vi "Choose Elevator Load Position.vi"(9 "Have Trashcan?":bool, 10 "Presets":T1, 11 "Command":T2) -> (3 "Elevator Position":dbl)   [LabVIEW 2014]
uses:
  Elevator Command.ctl
  Common Code/Elevator Presets.ctl
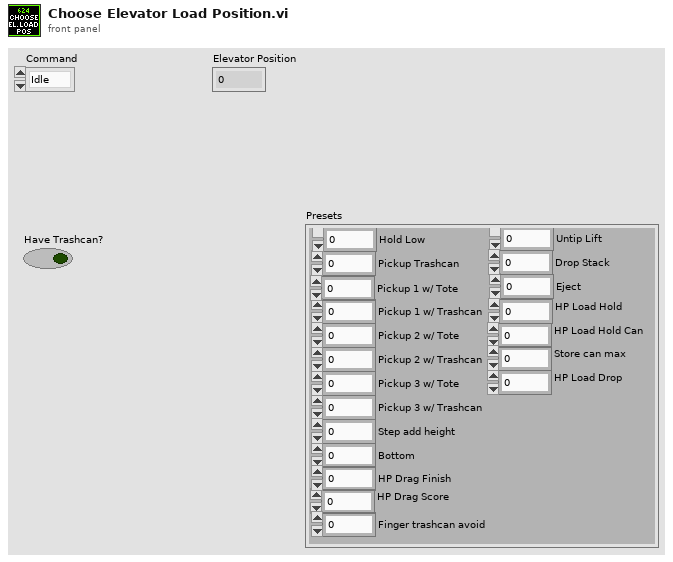
[diagram p1: front panel]
types:
  T1 = typedef "Elevator Presets.ctl" = cluster{"Pickup 2 w/ Tote":sgl, "Pickup 2 w/ Trashcan":sgl, "Pickup 3 w/ Tote":sgl, "Pickup 3 w/ Trashcan":sgl, "Bottom":sgl, "Pickup 1 w/ Tote":sgl, "Pickup Trashcan":sgl, "Pickup 1 w/ Trashcan":sgl, "Eject":sgl, "Hold Low":sgl, "Step add height":sgl, "Untip Lift":dbl, "Drop Stack":dbl, "HP Load Hold":dbl, "HP Load Drop":dbl, "HP Load Hold Can":dbl, "Store can max":dbl, "HP Drag Score":dbl, "HP Drag Finish":dbl, "Finger trashcan avoid":dbl}
  T2 = typedef "Elevator Command.ctl" = enum16{"Idle", "Load 1", "Load 2", "Load 3", "Drop Stack", "Eject Stack", "Untip Trashcan", "Load Trashcan", "HP Load", "HP Score"}
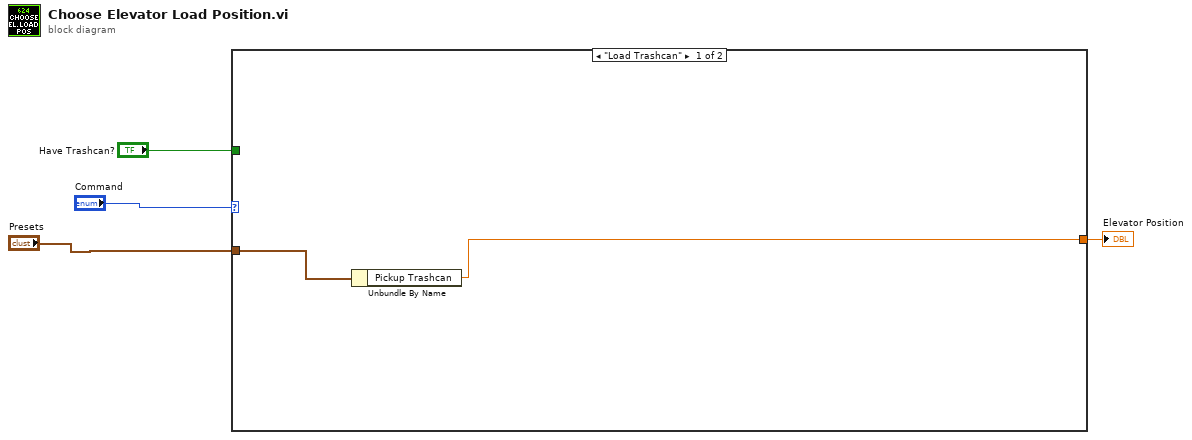
[diagram p0: block diagram]
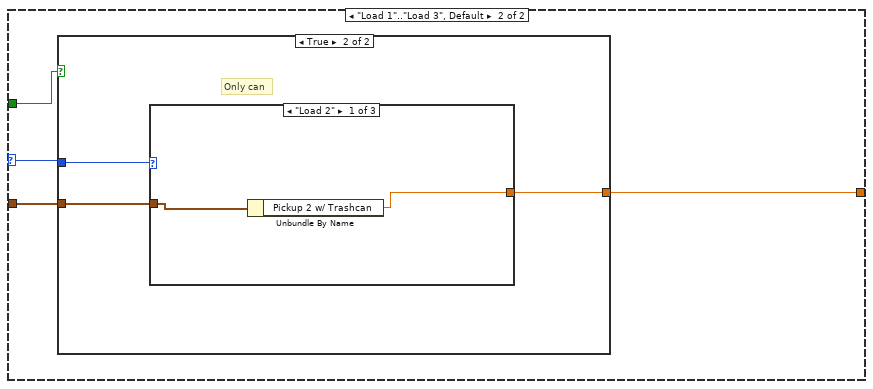
[diagram p2: hidden frame]
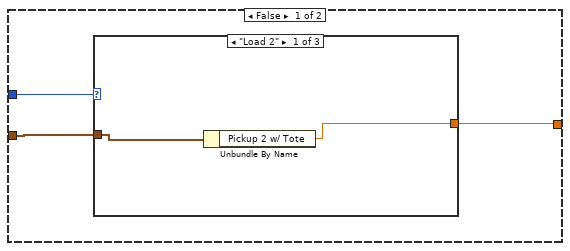
[diagram p3: hidden frame]
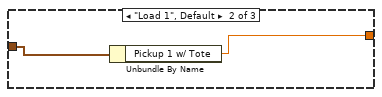
[diagram p4: hidden frame]
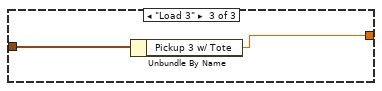
[diagram p5: hidden frame]
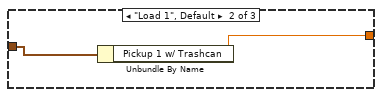
[diagram p6: hidden frame]
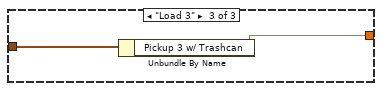
[diagram p7: hidden frame]
diagram:
  n1 = case shown="\"Load Trashcan\"" "Command" {
    selector: "Command" -> [_ w9]
    tunnel: "Presets" -> [w6 w10]
    tunnel: [w5 w8] -> w3
    tunnel: "Have Trashcan?" -> [_ w7]
    frame "Load Trashcan" {
      n2 = Unbundle By Name(w6) -> ("Pickup Trashcan"=w5:sgl)
    }
    frame "Load 1".."Load 3", Default {
      n3 = case shown="True" w7 {
        tunnel: w10 -> [w13 w22]
        tunnel: w9 -> [w12 w21]
        tunnel: [w11 w20] -> w8
        frame False {
          n4 = case shown="\"Load 2\"" w12 {
            tunnel: w13 -> [w15 w17 w19]
            tunnel: [w14 w16 w18] -> w11
            frame "Load 2" {
              n5 = Unbundle By Name(w15) -> ("Pickup 2 w/ Tote"=w14:sgl)
            }
            frame "Load 1", Default {
              n6 = Unbundle By Name(w17) -> ("Pickup 1 w/ Tote"=w16:sgl)
            }
            frame "Load 3" {
              n7 = Unbundle By Name(w19) -> ("Pickup 3 w/ Tote"=w18:sgl)
            }
          }
        }
        frame True {
          # "Only can"
          n8 = case shown="\"Load 2\"" w21 {
            tunnel: w22 -> [w24 w26 w28]
            tunnel: [w23 w25 w27] -> w20
            frame "Load 2" {
              n9 = Unbundle By Name(w24) -> ("Pickup 2 w/ Trashcan"=w23:sgl)
            }
            frame "Load 1", Default {
              n10 = Unbundle By Name(w26) -> ("Pickup 1 w/ Trashcan"=w25:sgl)
            }
            frame "Load 3" {
              n11 = Unbundle By Name(w28) -> ("Pickup 3 w/ Trashcan"=w27:sgl)
            }
          }
        }
      }
    }
  }
  "Elevator Position" <- w3
